vi "labview_data_publisher.vi"(1 "Cluster":T1) -> ()   [LabVIEW 2024]
uses:
  <vilib>/RTI DDS Toolkit/Types/RTI DDS Advanced Writer Configuration.ctl
  <vilib>/RTI DDS Toolkit/Library/LVDDS_library.lvlib
panel:
  in  "Advanced Writer Configuration":T2={"typeName"="octa_ros::msg::dds_::Labviewdata_", "keyName"="", "domainParticipantQoSProfile"="", "dataWriterQoSProfile"="", "forceArrayMapping?"=FALSE, "forceUnboundedString?"=FALSE}
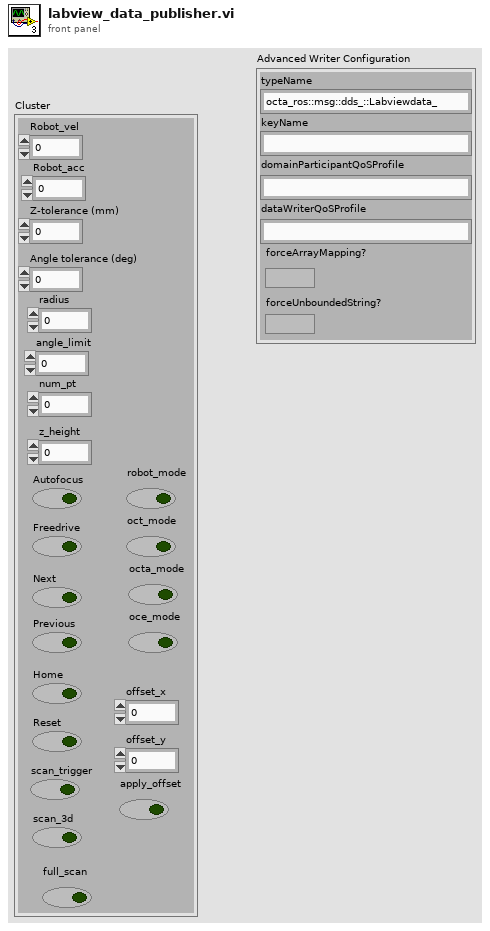
[diagram p1: front panel]
types:
  T1 = cluster{"Robot_vel":dbl, "Robot_acc":dbl, "Z-tolerance (mm)":dbl, "Angle tolerance (deg)":dbl, "radius":dbl, "angle_limit":dbl, "num_pt":i32, "z_height":dbl, "Autofocus":bool, "Freedrive":bool, "Next":bool, "Previous":bool, "Home":bool, "Reset":bool, "scan_trigger":bool, "scan_3d":bool, "full_scan":bool, "robot_mode":bool, "oct_mode":bool, "octa_mode":bool, "oce_mode":bool, "offset_x":dbl, "offset_y":dbl, "apply_offset":bool}
  T2 = typedef "LVDDS_library.lvlib/RTI DDS Advanced Writer Configuration.ctl" = cluster{"typeName":string, "keyName":string, "domainParticipantQoSProfile":string, "dataWriterQoSProfile":string, "forceArrayMapping?":bool, "forceUnboundedString?":bool}
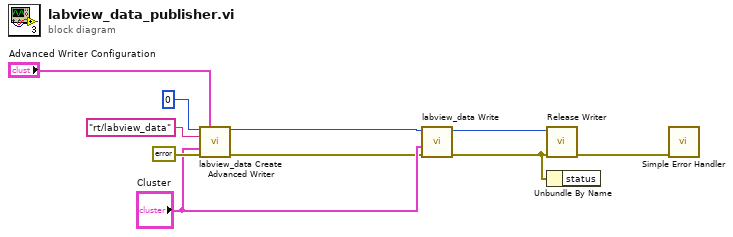
[diagram p0: block diagram]
diagram:
  n1 = call "labview_data Create Advanced Writer.vi"("Domain Id"=u32 0, "Advanced Writer Configuration"="Advanced Writer Configuration", "Topic Name"="rt/labview_data", "MyComplexType type"="Cluster", "error in (no error)"=errorcluster {"status"=FALSE, "code"=0, "source"=""}) -> ("DDS Object Ref"=w5:u64, "error out"=w4:errorcluster)  [unwired: 9 in]
  n2 = call "labview_data Write.vi"("error in (no error)"=w4, "MyComplexType"="Cluster", "DDS Object Ref in"=w5) -> ("error out"=w9:errorcluster, "DDS Object Ref out"=w6:u64)  [unwired: 7 in]
  n3 = call <vilib>:"Release Writer.vi"("error in (no error)"=w9, "DDS Object Ref"=w6) -> ("error out"=w8:errorcluster)  [unwired: 9 in]
  n4 = Unbundle By Name(w9) -> ()  [unwired: 1 out]
  n5 = call <vilib>:"Simple Error Handler.vi"("error in (no error)"=w8) -> ()  [unwired: 4 in, 5 out]
